vi "Autophase.vi"(8 "error in (no error)":errorcluster, 9 "Boolean":bool, 10 "Results":T1 {"Results (Dictionary)"."value" format="%#_6p"}, 11 "Instrument.DAQ in":refnum<class "Instrument.DAQ.lvclass">) -> (0 "error out":errorcluster, 3 "Instrument.DAQ out":refnum<class "Instrument.DAQ.lvclass">)   [LabVIEW 2019, in "Instrument.Lockin.lvlib" / "Instrument.DAQ.lvclass"]
uses:
  Instrument.DAQ.lvclass
  Typedefs/Results--Cluster.ctl
  Instrument.Lockin/Typedefs/Results Type--Enum.ctl
  Instrument.DAQ.lvclass/Instrument.DAQ.ctl
  <vilib>/addons/control/pid/pid.llb/PID (DBL Array).vi
  Instrument.Lockin/Instrument.Lockin.lvclass
  <vilib>/addons/control/pid/NI_PID_pid.lvlib
  <vilib>/addons/control/pid/pid.llb/PID Control Input Filter (DBL).vi
panel:
  out "output":dbl[](array[numeric]) format="%.2f"
  in  "D":dbl=0.019999999999999997 format="%.3f"
  in  "I":dbl=0.6 format="%.3f"
  in  "P":dbl=0.5 format="%.2f"
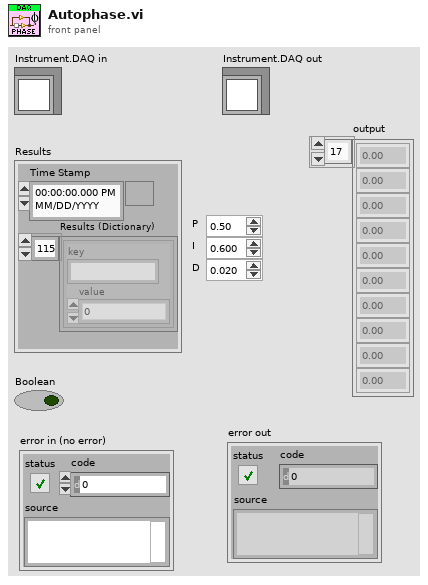
[diagram p1: front panel]
types:
  T1 = typedef "Instrument.Lockin.lvlib/Instrument.DAQ.lvclass/Results--Cluster.ctl" = cluster{"Time Stamp":timestamp, "Results (Dictionary)":cluster{"key":string, "value":dbl}[]}
  T2 = cluster{"proportional gain (Kc)":dbl, "integral time (Ti, min)":dbl, "derivative time (Td, min)":dbl}
  T3 = typedef "Instrument.Lockin.lvlib/Instrument.Lockin.lvclass/Results Type--Enum.ctl" = enum16{"X", "Y", "R", "Theta", "Mean"}
  T4 = typedef "Instrument.Lockin.lvlib/Instrument.DAQ.lvclass/AO.Channel--Cluster--Array.ctl" = T5[]
  T5 = typedef "Instrument.Lockin.lvlib/Instrument.DAQ.lvclass/AO.Channel--Cluster.ctl" = cluster{"Enable?":bool, "Channel":i32, "Amplitude":dbl, "Offset":dbl, "Frequency":dbl, "Phase":dbl, "Function":T6, "Sweeping?":bool, "Limit AC":bool, "Limit DC?":bool}
  T6 = typedef "Instrument.Lockin.lvlib/Instrument.DAQ.lvclass/AO.Channel.Function--Enum.ctl" = enum16{"Sine", "Triangle", "Square"}
  T7 = cluster{"proportional gain (Kc)":dbl, "integral time (Ti, min)":dbl, "derivative time (Td, min)":dbl}[]
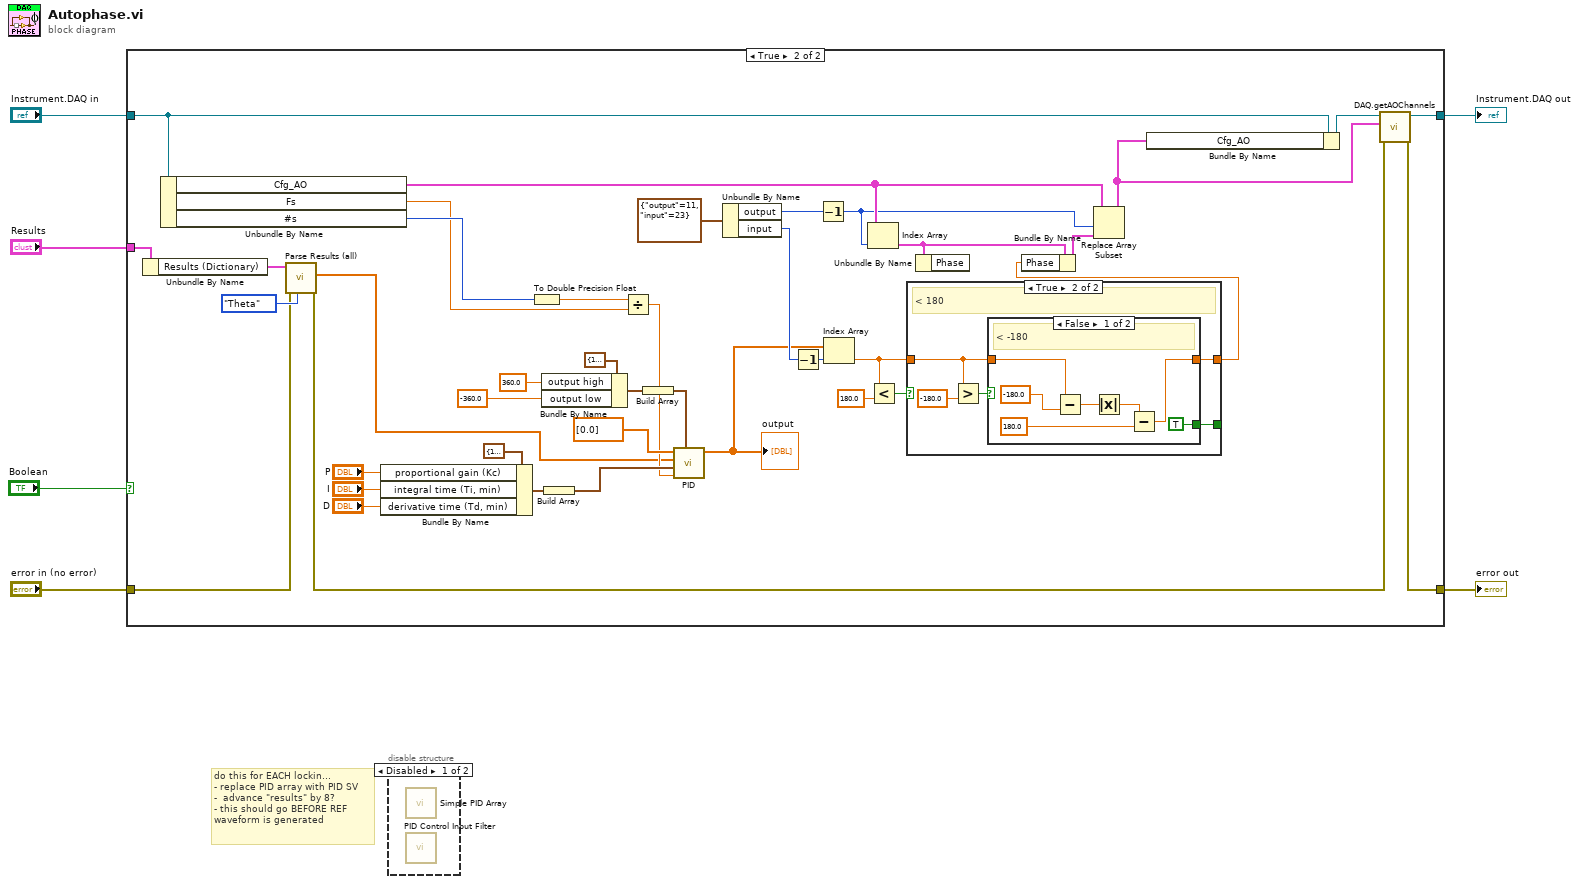
[diagram p0: block diagram]
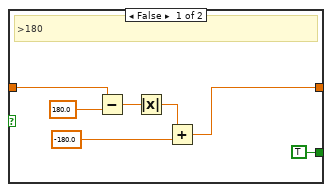
[diagram p3: hidden frame]
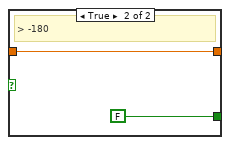
[diagram p4: hidden frame]
diagram:
  # "do this for EACH lockin...\n- replace PID array with PID SV\n-  advance \"results\" by 8?\n- this should go BEFORE REF\nwaveform is generated"
  n1 = case shown="True" "Boolean" {
    tunnel: "Instrument.DAQ in" -> [w8 w9]
    tunnel: "Results" -> [_ w48]
    tunnel: "error in (no error)" -> [w7 w10]
    tunnel: [w8 w47] -> w3
    tunnel: [w7 w11] -> w2
    frame False {
    }
    frame True {
      n2 = Unbundle By Name(w48) -> ("Results (Dictionary)"=w46:cluster{"key":string, "value":dbl}[])
      n3 = Unbundle By Name(w9) -> ("Cfg_AO"=w30:T4, "Fs"=w20:dbl, "#s"=w21:i32)
      n4 = call "Parse Results (all).vi"("Type"=Results_Type--Enum."Theta", "error in (no error)"=w10, "Results (Dictionary)"=w46) -> ("error out"=w43:errorcluster, "Data"=w12:dbl[])  [unwired: 5 in, 2 out]
      n5 = Bundle By Name(cluster=T2 {"proportional gain (Kc)"=1.0, "integral time (Ti, min)"=0.01, "derivative time (Td, min)"=0.0} ("PID gains"), "proportional gain (Kc)"="P", "integral time (Ti, min)"="I", "derivative time (Td, min)"="D") -> (w36:T2)
      n6 = To Double Precision Float(number=w21) -> (double precision float=w13:dbl)
      n7 = Bundle By Name(cluster=cluster{"output high":dbl, "output low":dbl} {"output high"=100.0, "output low"=-100.0} ("output range"), "output high"=360.0, "output low"=-360.0) -> (w37:cluster{"output high":dbl, "output low":dbl})
      n8 = Build Array(w36) -> (w32:T7)
      n9 = Divide(x=w13, y=w20) -> (x/y=w19:dbl)
      n10 = Build Array(w37) -> (w28:cluster{"output high":dbl, "output low":dbl}[])
      n11 = call-poly <vilib>:"PID.vi"("output range"=w28, "dt (s)"=w19, "PID gains"=w32, "process variable"=w12, "setpoint"=dbl[] [0.0]) -> ("output"=w18:dbl[])  [unwired: 5 in, 1 out]
      "output" <- w18
      n12 = Unbundle By Name(cluster{"output":i32, "input":i32} {"output"=11, "input"=23}) -> ("output"=w26:i32, "input"=w25:i32)
      n13 = Decrement(x=w25) -> (x-1=w24:i32)
      n14 = Decrement(x=w26) -> (x-1=w23:i32)
      n15 = Index Array(array=w18, index=w24) -> (element=w15:dbl)
      n16 = Index Array(array=w30, index=w23) -> (element=w31:T5)
      n17 = Less?(x=w15, y=180.0) -> (x < y?=w16:bool)
      n18 = case shown="True" w16 {
        tunnel: w15 -> [w51 w57]
        tunnel: [w50 w58] -> w14
        tunnel: [TRUE w56] -> _
        frame False {
          # ">180"
          n19 = Subtract(x=w51, y=180.0) -> (x-y=w54:dbl)
          n20 = Absolute Value(x=w54) -> (abs(x)=w53:dbl)
          n21 = Add(x=w53, y=-180.0) -> (x+y=w50:dbl)
        }
        frame True {
          # "< 180"
          n22 = Greater?(x=w57, y=-180.0) -> (0:w60:bool)
          n23 = case shown="False" w60 {
            tunnel: [w62 w69] -> w58
            tunnel: w57 -> [w63 w69]
            tunnel: [TRUE FALSE] -> w56
            frame False {
              # "< -180"
              n24 = Subtract(x=w63, y=-180.0) -> (x-y=w66:dbl)
              n25 = Absolute Value(x=w66) -> (abs(x)=w65:dbl)
              n26 = Subtract(x=w65, y=180.0) -> (x-y=w62:dbl)
            }
            frame True {
              # "> -180"
            }
          }
        }
      }
      n27 = Unbundle By Name(w31) -> ()  [unwired: 1 out]
      n28 = Bundle By Name(cluster=w31, "Phase"=w14) -> (w29:T5)
      n29 = Replace Array Subset(array=w30, new element=w29, index=w23) -> (w22:T4)
      n30 = Bundle By Name(cluster=w9, "Cfg_AO"=w22) -> (w44:refnum<class "Instrument.DAQ.lvclass">)
      n31 = call "DAQ.getAOChannels.vi"("error in (no error)"=w43, "Channels: AO"=w22, "Instrument.DAQ"=w44) -> ("error out"=w11:errorcluster, "Instrument.DAQ out"=w47:refnum<class "Instrument.DAQ.lvclass">)  [unwired: 7 in]
    }
  }
  "Instrument.DAQ out" <- w3
  "error out" <- w2
  n32 = disable-structure shown="Disabled" {
    frame Disabled {
      n33 = call "Simple PID Array.vi"() -> ()  [unwired: 11 in, 1 out]
      n34 = call-poly <vilib>:"PID Control Input Filter.vi"() -> ()  [unwired: 5 in, 1 out]
    }
    frame Enabled {
    }
  }
